vi "PositionControlCANTest.vi"() -> ()   [LabVIEW 2009, in "Test.lvlib"]
uses:
  CAN/SubVIs/CAN Jaguar Control Mode.ctl
  Test.lvlib
  OWNCAN.lvlib
  CAN.lvlib
panel:
  in  "D":dbl
  in  "I":dbl
  in  "P":dbl
  out "error out pid":errorcluster
  in  "Set PID":bool
  in  "Maximum Output Voltage":dbl=5.0
  out "error out hb":errorcluster
  out "error out close":errorcluster
  in  "Output Right":dbl
  in  "Output Left":dbl
  out "error out set out":errorcluster
  in  "stop":bool
  in  "Execute":bool
  in  "Control Mode":T1=enum."Position"
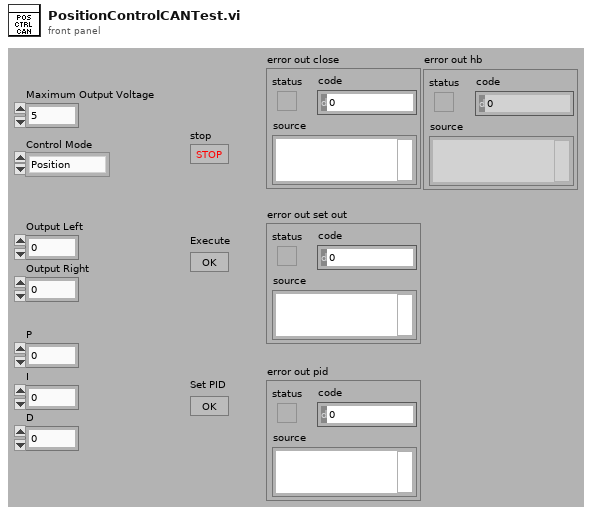
[diagram p1: front panel]
types:
  T1 = typedef "CAN.lvlib/CAN Jaguar Control Mode.ctl" = enum16{"Percent VBus", "Speed", "Position", "Current"}
  T2 = typedef "OWNCAN.lvlib/CAN Jaguars Ref.ctl" = cluster{"CAN Jaguar Ref Left":T3, "CAN Jaguar Ref Right":T3}
  T3 = typedef "CAN.lvlib/CAN Jaguar Ref.ctl" = cluster{"Device Number":u8, "Control Mode":T1, "Inverted":bool, "Semaphore":T4, "Max Vout":dbl, "DevStatus":errorcluster}
  T4 = typedef "Semaphore RefNum" = refnum<k1>
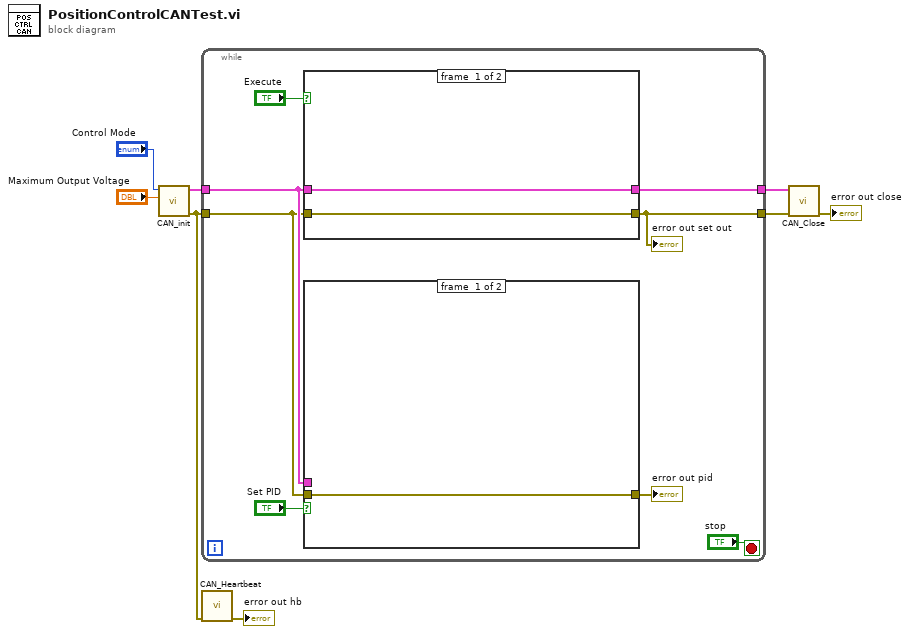
[diagram p0: block diagram]
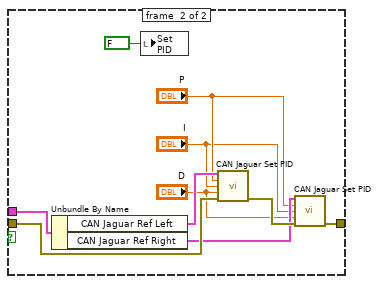
[diagram p2: hidden frame]
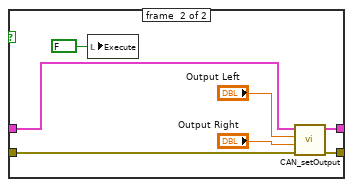
[diagram p3: hidden frame]
diagram:
  n1 = call "CAN_init.vi"("Maximum Output Voltage"="Maximum Output Voltage", "Control Mode"="Control Mode") -> ("error out"=w7:errorcluster, "CAN Jaguars Ref"=w5:T2)  [unwired: 6 in]
  n2 = while {
    tunnel: w7 -> [w9]
    tunnel: [w14] -> w6
    tunnel: w5 -> [w10]
    tunnel: [w13] -> w4
    stop <- "stop" stop-if-true
    n3 = case shown="True" "Execute" {
      tunnel: w9 -> [w29 w35]
      tunnel: [w29 w34] -> w14
      tunnel: w10 -> [w28 w31]
      tunnel: [w28 w30] -> w13
      frame #0 {
      }
      frame #1 {
        n4 = local write "Execute"(FALSE ("OK Button")) -> ()
        n5 = call "CAN_setOutput.vi"("error in (no error)"=w35, "Output Right"="Output Right", "Output Left"="Output Left", "CAN Jaguars Ref"=w31) -> ("error out"=w34:errorcluster, "CAN Jaguars Ref out"=w30:T2)  [unwired: 6 in]
      }
    }
    "error out set out" <- w14
    n6 = case shown="True" "Set PID" {
      tunnel: w9 -> [w17 w24]
      tunnel: [w17 w22] -> w11
      tunnel: w10 -> [_ w26]
      frame #0 {
      }
      frame #1 {
        n7 = Unbundle By Name(w26) -> ("CAN Jaguar Ref Left"=w25:T3, "CAN Jaguar Ref Right"=w21:T3)
        n8 = local write "Set PID"(FALSE ("OK Button")) -> ()
        n9 = call "CAN Jaguar Set PID.vi"("CAN Jaguar Ref"=w25, "P"="P", "I"="I", "D"="D", "error in (no error)"=w24) -> ("error out"=w23:errorcluster)  [unwired: 9 in, 1 out]
        n10 = call "CAN Jaguar Set PID.vi"("CAN Jaguar Ref"=w21, "P"="P", "I"="I", "D"="D", "error in (no error)"=w23) -> ("error out"=w22:errorcluster)  [unwired: 9 in, 1 out]
      }
    }
    "error out pid" <- w11
  }
  n11 = call "CAN_Heartbeat.vi"("error in"=w7) -> ("error out"=→"error out hb":errorcluster)  [unwired: 10 in]
  n12 = call "CAN_Close.vi"("error in"=w6, "CAN Jaguars Ref"=w4) -> ("error out"=→"error out close":errorcluster)  [unwired: 9 in]
